vi "UpdateGUIconnectionTable.vi"(8 "error in (no error)":errorcluster, 11 "TCP_Server in":refnum<class "TCP_Server.lvclass">) -> (0 "error out":errorcluster, 3 "TCP_Server out":refnum<class "TCP_Server.lvclass">)   [LabVIEW 2023, in "TCP_Server.lvlib" / "TCP_Server.lvclass"]
uses:
  TCP_Server.lvclass
  TCP_Server.lvclass/TCP_Server.ctl
  TCP_serverGUI/TCP_serverGUI Messages/UpdateConnectionsListbox Msg/UpdateConnectionsListbox Msg.lvclass
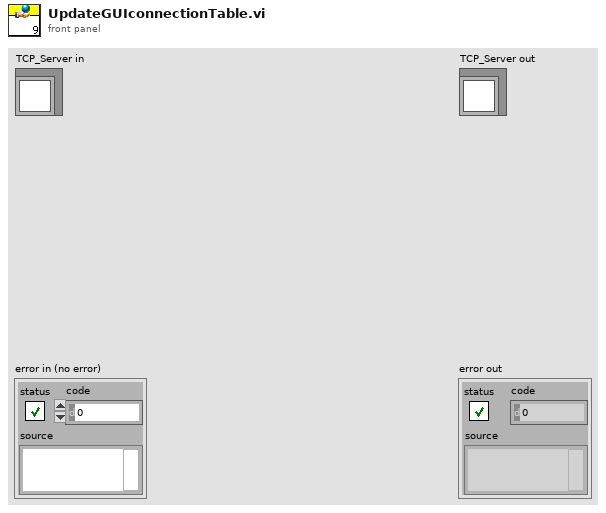
[diagram p1: front panel]
types:
  T1 = typedef "TCP_Server.lvlib/ServerConnection.ctl" = cluster{"Connection Handlers's Enqueuer":refnum<class "Message Enqueuer.lvclass">, "Connection Window's Enqueuer":refnum<class "Message Enqueuer.lvclass">, "Connection Information":T2}
  T2 = typedef "TCP_Listener.lvlib/ConnectionInformation.ctl" = cluster{"Connection number":i32, "Remote Address":string, "Remote Port":u16, "Connection ID":refnum<k5>}
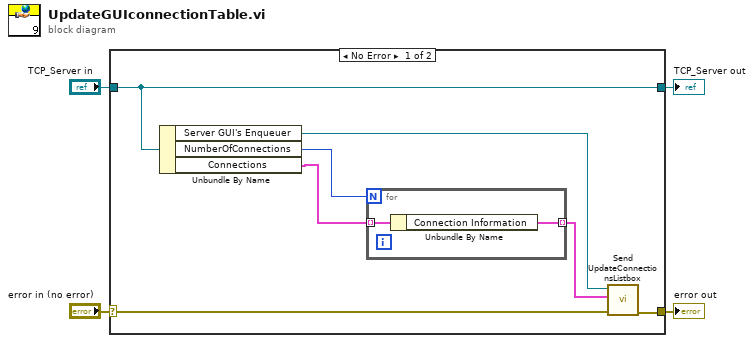
[diagram p0: block diagram]
diagram:
  n1 = case shown="No Error" "error in (no error)" {
    selector: "error in (no error)" -> [w6 w15]
    tunnel: [w5 w15] -> w3
    tunnel: [w11 w14] -> w1
    tunnel: "TCP_Server in" -> [w11 w14]
    frame No Error {
      n2 = Unbundle By Name(w11) -> ("Server GUI's Enqueuer"=w7:refnum<class "Message Enqueuer.lvclass">, "NumberOfConnections"=w10:i32, "Connections"=w9:T1[])
      n3 = for {
        N: w10 -> [_]
        tunnel: w9 -> [w13] mode=indexing
        tunnel: [w12] -> w8 mode=indexing
        n4 = Unbundle By Name(w13) -> ("Connection Information"=w12:T2)
      }
      n5 = call "Send UpdateConnectionsListbox.vi"("error in (no error)"=w6, "Connections"=w8, "Message Enqueuer"=w7) -> ("error out"=w5:errorcluster)  [unwired: 7 in, 1 out]
    }
    frame Error {
    }
  }
  "error out" <- w3
  "TCP_Server out" <- w1
